vi "Generic command handler.vi"(8 "error in (no error)":errorcluster, 10 "Message in":refnum<class "GenericMessage.lvclass">, 11 "ImageStack in":refnum<class "ImageStack.lvclass">) -> (0 "error out":errorcluster, 2 "value":string, 3 "ImageStack out":refnum<class "ImageStack.lvclass">)   [LabVIEW 2012, in "ImageStack.lvclass"]
doc: "The generic_command_handler processes the command 'generic'. Commands which are not part of the predefined list of commands fall under the 'generic' command for special activity."
uses:
  ImageStack.lvclass
  <vilib>/Distrio/Murmex/GenericMessage/GenericMessage.lvclass
  <vilib>/Distrio/Murmex/Murmex/Murmex.lvclass
  ImageStack.lvclass/ImageStack.ctl
  <vilib>/Distrio/Murmex/Message/Message.lvclass
panel:
  # "This method is called when the GENERIC\ntrigger is sent. \n\nOverride this method when your component needs to\nrespond to this trigger. \n\nCall parent for proper implementation"
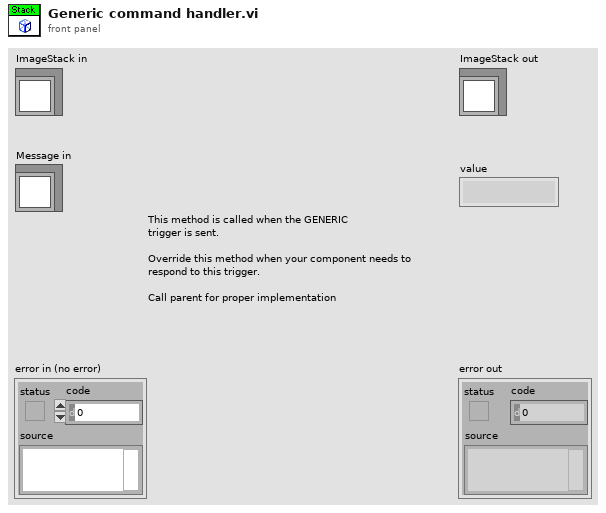
[diagram p1: front panel]
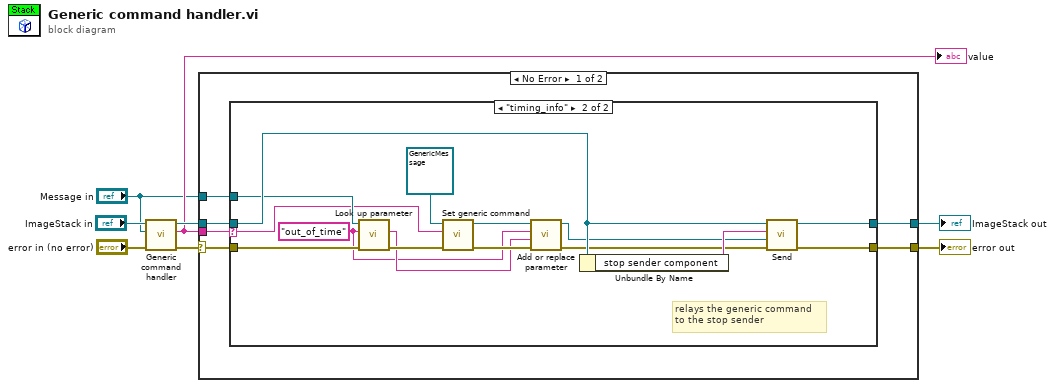
[diagram p0: block diagram]
diagram:
  n1 = call-parent "Generic command handler.vi"("error in (no error)"="error in (no error)", "Message in"="Message in", "Murmex in"="ImageStack in") -> ("error out"=w6:errorcluster, "value"=w2:string, "Murmex out"=w5:refnum<class "ImageStack.lvclass">)  [unwired: 6 in]
  "value" <- w2
  n2 = case shown="No Error" w6 {
    selector: w6 -> [w12 w32]
    tunnel: w5 -> [w13 w33]
    tunnel: w2 -> [w14 _]
    tunnel: [w11 w33] -> w4
    tunnel: [w10 w32] -> w3
    tunnel: "Message in" -> [w9 _]
    frame No Error {
      n3 = case shown="\"timing_info\"" w14 {
        selector: w14 -> [_ w21]
        tunnel: w13 -> [w16 w28]
        tunnel: w12 -> [w15 w27]
        tunnel: [w16 w31] -> w11
        tunnel: [w15 w30] -> w10
        tunnel: w9 -> [_ w26]
        frame Default {
        }
        frame "timing_info" {
          w18 = "out_of_time" ("name")
          # "relays the generic command\nto the stop sender"
          n4 = call <vilib>:"Look up parameter.vi"("error in (no error)"=w27, "name"=w18, "Message in"=w26) -> ("error out"=w24:errorcluster, "key"=w19:string)  [unwired: 5 in, 2 out]
          n5 = call <vilib>:"Set generic command.vi"("error in (no error)"=w24, "generic command"=w21, "GenericMessage in"=refnum<class "GenericMessage.lvclass"> refnum ("Distrio Murmex 1.2:GenericMessage")) -> ("error out"=w23:errorcluster, "GenericMessage out"=w20:refnum<class "GenericMessage.lvclass">)  [unwired: 7 in]
          n6 = call <vilib>:"Add or replace parameter.vi"("error in (no error)"=w23, "value"=w19, "name"=w18, "Message in"=w20) -> ("error out"=w25:errorcluster, "Message out"=w17:refnum<class "GenericMessage.lvclass">)  [unwired: 6 in]
          n7 = Unbundle By Name(w28) -> ("stop sender component"=w29:string)
          n8 = call <vilib>:"Send.vi"("error in (no error)"=w25, "Message"=w17, "recipient"=w29, "Murmex in"=w28) -> ("error out"=w30:errorcluster, "Murmex out"=w31:refnum<class "ImageStack.lvclass">)  [unwired: 6 in]
        }
      }
    }
    frame Error {
    }
  }
  "error out" <- w3
  "ImageStack out" <- w4
